vi "marshalling.vi"(8 "error in (no error)":errorcluster, 10 "Variant":variant, 11 "Serializer.Base64 in":refnum<class "Serializer.Base64.lvclass">) -> (0 "error out":errorcluster, 2 "String":string, 3 "Serializer.Base64 out":refnum<class "Serializer.Base64.lvclass">)   [LabVIEW 2019, in "OpenSerializer.base64.lvlib" / "Serializer.Base64.lvclass"]
uses:
  Serializer.Base64.lvclass
  Base64_CharSet.vi
  <vilib>/LabVIEW Open Source Project/OpenSerializer/Serializer.FlattenedString/Serializer.FlattenedString.lvclass
  OpenSerializer.base64.lvlib
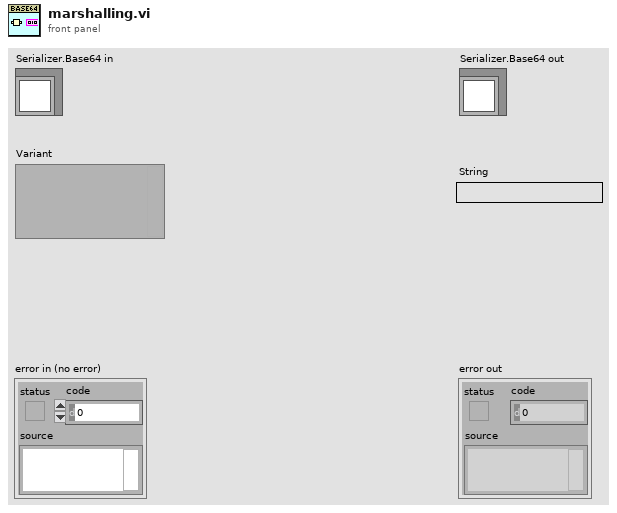
[diagram p1: front panel]
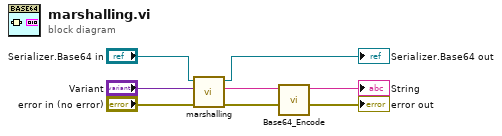
[diagram p0: block diagram]
diagram:
  n1 = call-parent "marshalling.vi"("error in (no error)"="error in (no error)", "Variant"="Variant", "Serializer in"="Serializer.Base64 in") -> ("error out"=w4:errorcluster, "String"=w2:string, "Serializer out"=→"Serializer.Base64 out":refnum<class "Serializer.Base64.lvclass">)  [unwired: 6 in]
  n2 = call "Base64_Encode.vi"("error in (no error)"=w4, "String"=w2) -> ("error out"=→"error out":errorcluster, "Encoded String"=→"String":string)  [unwired: 8 in]
